vi "test.ini_to_toml.vi"() -> ()   [LabVIEW 2020]
uses:
  <vilib>/addons/_JKI Toolkits/Caraya/classes/Test/Test.lvclass
panel:
  out "TOML (Expected) 2":string="[booleans]\nfoo = true\nbar = false\nbuz = true\nbaz = false"
  out "TOML (Expected)":string="[booleans]\nfoo = true\nbar = false\nbuz = true\nbaz = false"
  out "Actual Converted TOML out":string="[booleans]\nfoo = true\nbar = false\nbuz = true\nbaz = false"
  out "error out":errorcluster
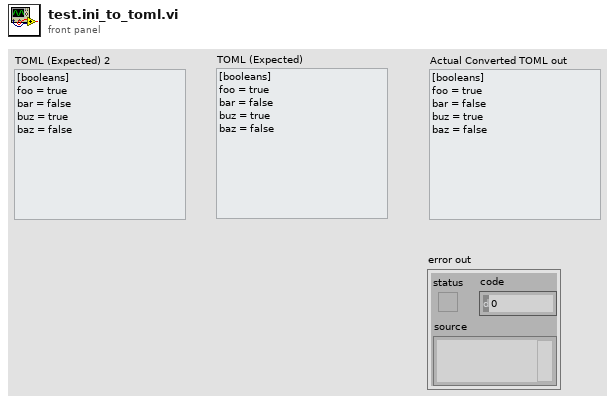
[diagram p1: front panel]
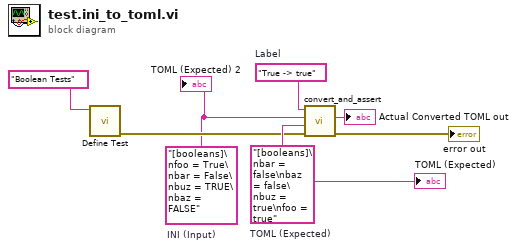
[diagram p0: block diagram]
diagram:
  w5 = "[booleans]\nbar = false\nbaz = false\nbuz = true\nfoo = true"  # TOML (Expected)
  w1 = "[booleans]\nfoo = True\nbar = False\nbuz = TRUE\nbaz = FALSE"  # INI (Input)
  w6 = "True -> true"  # Label
  n1 = call <vilib>:"Define Test.vi"("Label (VI Title)"="Boolean Tests") -> ("error out"=w4:errorcluster)  [unwired: 10 in]
  n2 = call "convert_and_assert.vi"("error in (no error)"=w4, "Config String (\"\")"=w5, "Config String (\"\") 2"=w1, "Label"=w6) -> ("error out"=→"error out":errorcluster, "converted toml out"=→"Actual Converted TOML out":string)  [unwired: 6 in]
  "TOML (Expected)" <- w5
  "TOML (Expected) 2" <- w1
